vi "CubeLiftControl.vi"(2 "Cube Lift Command":T3) -> (6 "CubeLiftOutput":T1 {"LiftControlMode" items=["PercentOutput"=0, "Position"=1, "Velocity"=2, "Current"=3, "Follower"=5, "MotionProfile"=6, "MotionMagic"=7, "MotionMagicArc"=8, "MotionProfileArc"=10, "Disabled"=15]})   [LabVIEW 2017]
uses:
  CubeLiftCommand.ctl
  RunMode.ctl
  CubeLiftOutput.ctl
  <vilib>/Rock Robotics/WPI/ThirdParty/Phoenix-LabVIEW/Motor Controller/Controls/CTRE_Phoenix_MotorControl_ControlMode.ctl
  SubsystemData/CubeLiftData/CubeLiftData.lvclass
  RobotSubsystem.lvclass
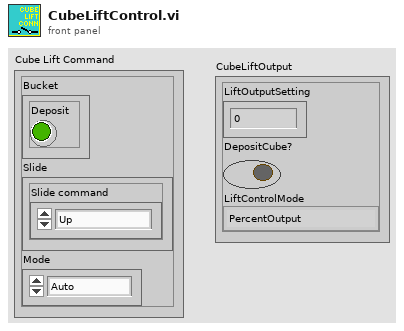
[diagram p1: front panel]
types:
  T1 = typedef "CubeLiftData.lvclass/CubeLiftOutput.ctl" = cluster{"LiftOutputSetting":dbl, "DepositCube?":bool, "LiftControlMode":T2}
  T2 = typedef "CTRE_Phoenix_MotorControl_ControlMode.ctl" = u16
  T3 = typedef "CubeLiftData.lvclass/CubeLiftCommand.ctl" = cluster{"Bucket":cluster{"Deposit":bool}, "Slide":cluster{"Slide command":enum16{"Up", "Down", "Stationary"}}, "Mode":T4}
  T4 = typedef "RobotSubsystem.lvclass/RunMode.ctl" = enum16{"Auto", "Teleop", "Disabled"}
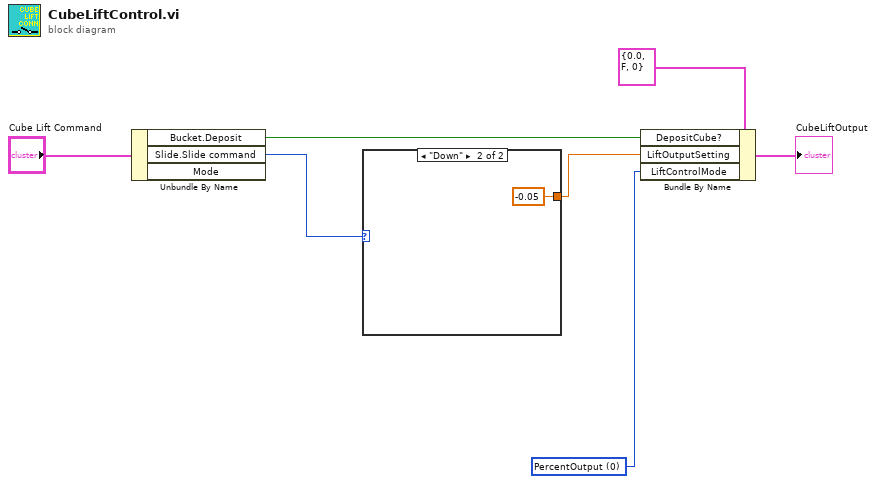
[diagram p0: block diagram]
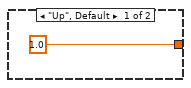
[diagram p2: hidden frame]
diagram:
  w4 = T2 0 items=["PercentOutput"=0, "Position"=1, "Velocity"=2, "Current"=3, "Follower"=5, "MotionProfile"=6, "MotionMagic"=7, "MotionMagicArc"=8, "MotionProfileArc"=10, "Disabled"=15] ("LiftControlMode")
  n1 = Unbundle By Name("Cube Lift Command") -> ("Bucket.Deposit"=w3:bool, "Slide.Slide command"=w2:enum16{"Up", "Down", "Stationary"})  [unwired: 1 out]
  n2 = case shown="\"Down\"" w2 {
    tunnel: [1.0 -0.05] -> w1
    frame "Up", Default {
    }
    frame "Down" {
    }
  }
  n3 = Bundle By Name(cluster=T1 {"LiftOutputSetting"=0.0, "DepositCube?"=FALSE, "LiftControlMode"=0} ("CubeLiftOutput 2"), "DepositCube?"=w3, "LiftOutputSetting"=w1, "LiftControlMode"=w4) -> (→"CubeLiftOutput":T1)
